vi "York DIHB - Data Capture.vi"() -> ()   [LabVIEW 2020]
doc: "VI used to capture strain gauge data from a Hopskinsons Bar experiment.\n\nOptionally, a calibration (lbs force vs. strain gauge output voltage correlation) can be applied to the measurement data. An interpolation/low pass filter algorith can be used to reduce signal noise.\n\nThe VI uses a queued message handler structure."
uses:
  Typedefs/Messages Cluster - Typedef.ctl
  Typedefs/Program State - Enum.ctl
  Typedefs/GUI Inputs Cluster - Typedef.ctl
  Typedefs/User Event - Enum.ctl
  Typedefs/Program Data - Typedef.ctl
  <vilib>/DAQmx/read.llb/DAQmx Read (Analog 1D Wfm NChan NSamp).vi
  <vilib>/Analysis/5stat.llb/RMS (DBL).vi
  <vilib>/DAQmx/configure/timing.llb/DAQmx Timing (Sample Clock).vi
  <vilib>/DAQmx/configure/trigger.llb/DAQmx Start Trigger (Analog Edge).vi
  <vilib>/DAQmx/miscellaneous.llb/DAQmx Fill In Error Info.vi
  <vilib>/DAQmx/create/channels.llb/DAQmx Create Channel (AI-Voltage-Basic).vi
  <vilib>/Utility/error.llb/Error Cluster From Error Code.vi
  <vilib>/ErrorRing/Error Ring.xnode
  <vilib>/Analysis/NI_AALPro.lvlib
panel:
  out "Projectile Velocity (m/s)":dbl
  out "First Pulse Data":waveform(dbl)(graph)
  out "Gates Graph":waveform(dbl)[](graph)
  out "Strain Gauge Graph":waveform(dbl)(graph)
  out "Warning Icon - Calibration":bool
  out "Warning Icon - Filepath":bool
  in  "Interpolation (Low Pass Filter)":i32
  in  "Calibration File (TXT TSV)":path
  out "File Save Progress":dbl(slide) scale=0.0..100.0
  in  "Filepath to Save Data (TSV)":path
  out "System Ready":bool
  in  "Ready Button":bool
  out "Millions of Samples":dbl
  out "Sample Rate (MHz)":dbl
  in  "Number of Samples":i32=1000000 format="%_3e"
  in  "Sample Rate (Hz)":dbl=2000000.0 format="%_3e"
  # "Instructions\n-Click the run arrow\n-Enter the desired sample rate, the number of samples\n  and the file name.\n-Click Ready\n-Pull the projectile backwards, using the string\n-Clear the impact area\n-Turn on the power switch\n-Push the fire switch\n\nNote: Zero time is time when the fire switch is pressed"
  # "Resolution Increase (bits)"
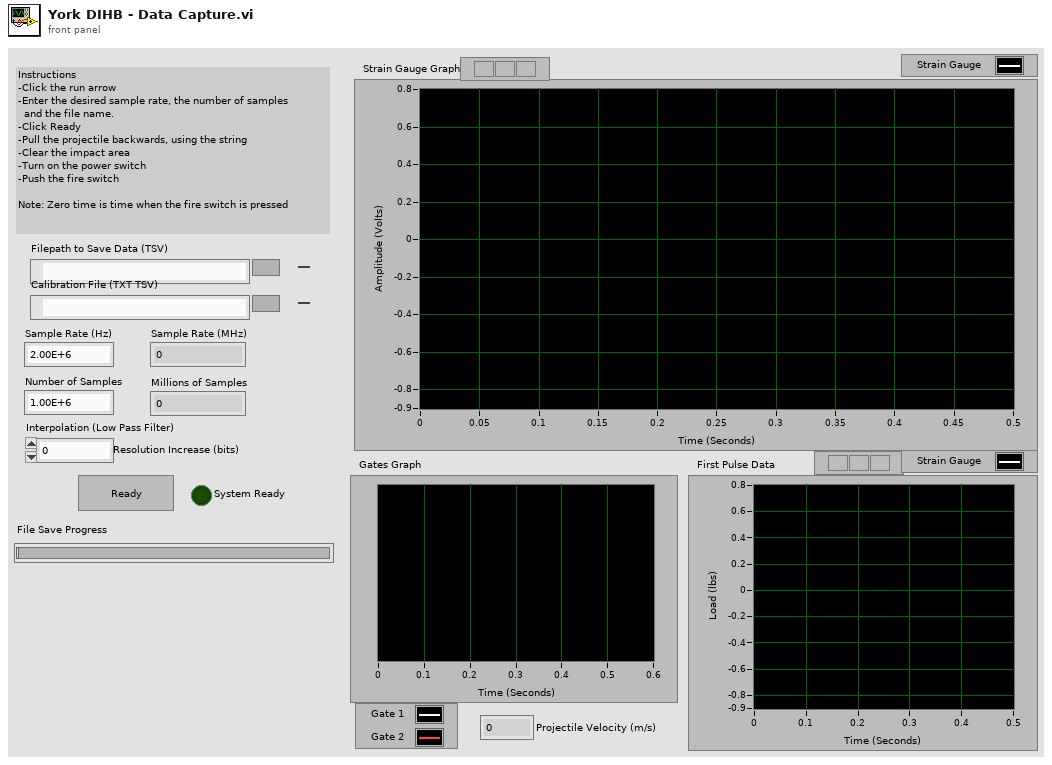
[diagram p1: front panel]
types:
  T1 = typedef "Program Data - Typedef.ctl" = cluster{"DAQmx Task Name":refnum<k21>, "Calibration Y - Load (lbs)":dbl[], "Calibration X - Strain Amplifier (V)":dbl[], "Calibration Slope (lbs/V)":dbl, "Calibration Intercept (lbs)":dbl, "Calibration Error":bool, "Gate 1 (V)":waveform(dbl), "Gate 2 (V)":waveform(dbl), "Strain (V)":waveform(dbl), "Projectile Velocity (m/s)":dbl, "Signal (V)":waveform(dbl), "Noise (V)":waveform(dbl), "Signal to noise ratio":dbl, "Pulse Start Time (ms)":dbl, "Calibrated Signal (lbs)":waveform(dbl), "Filtered Signal (V)":waveform(dbl), "Signal to noise ratio (filtered)":dbl}
  T2 = typedef "User Event - Enum.ctl" = enum16{"Shutdown"}
  T3 = typedef "Program State - Enum.ctl" = enum16{"Make Ready", "Calculate All", "Calculate Velocity", "Calculate Peak Start Time", "Calculate Calibrated Values", "Calculate Filtered Data", "Calculate SNR", "Capture Data", "Download Data", "Load Calibration", "GUI Update", "GUI Show Charts", "GUI Disable Controls", "GUI Enable Controls", "Save Data", "Save Filtered Data", "Save Calibrated Data", "Initialize", "Initialize DAQmx", "Shutdown"}
  T4 = typedef "Messages Cluster - Typedef.ctl" = cluster{"Program State":T3, "GUI Cluster":T5}
  T5 = typedef "GUI Inputs Cluster - Typedef.ctl" = cluster{"Sample Rate (Hz)":dbl, "Number of Samples":i32, "Ready Button":bool, "Filepath to Save Data":path, "Calibration File (TXT TSV)":path, "Interpolation (LP Filter)":dbl}
  T6 = enum8{"Enabled", "Disabled", "Disabled and Grayed Out"}
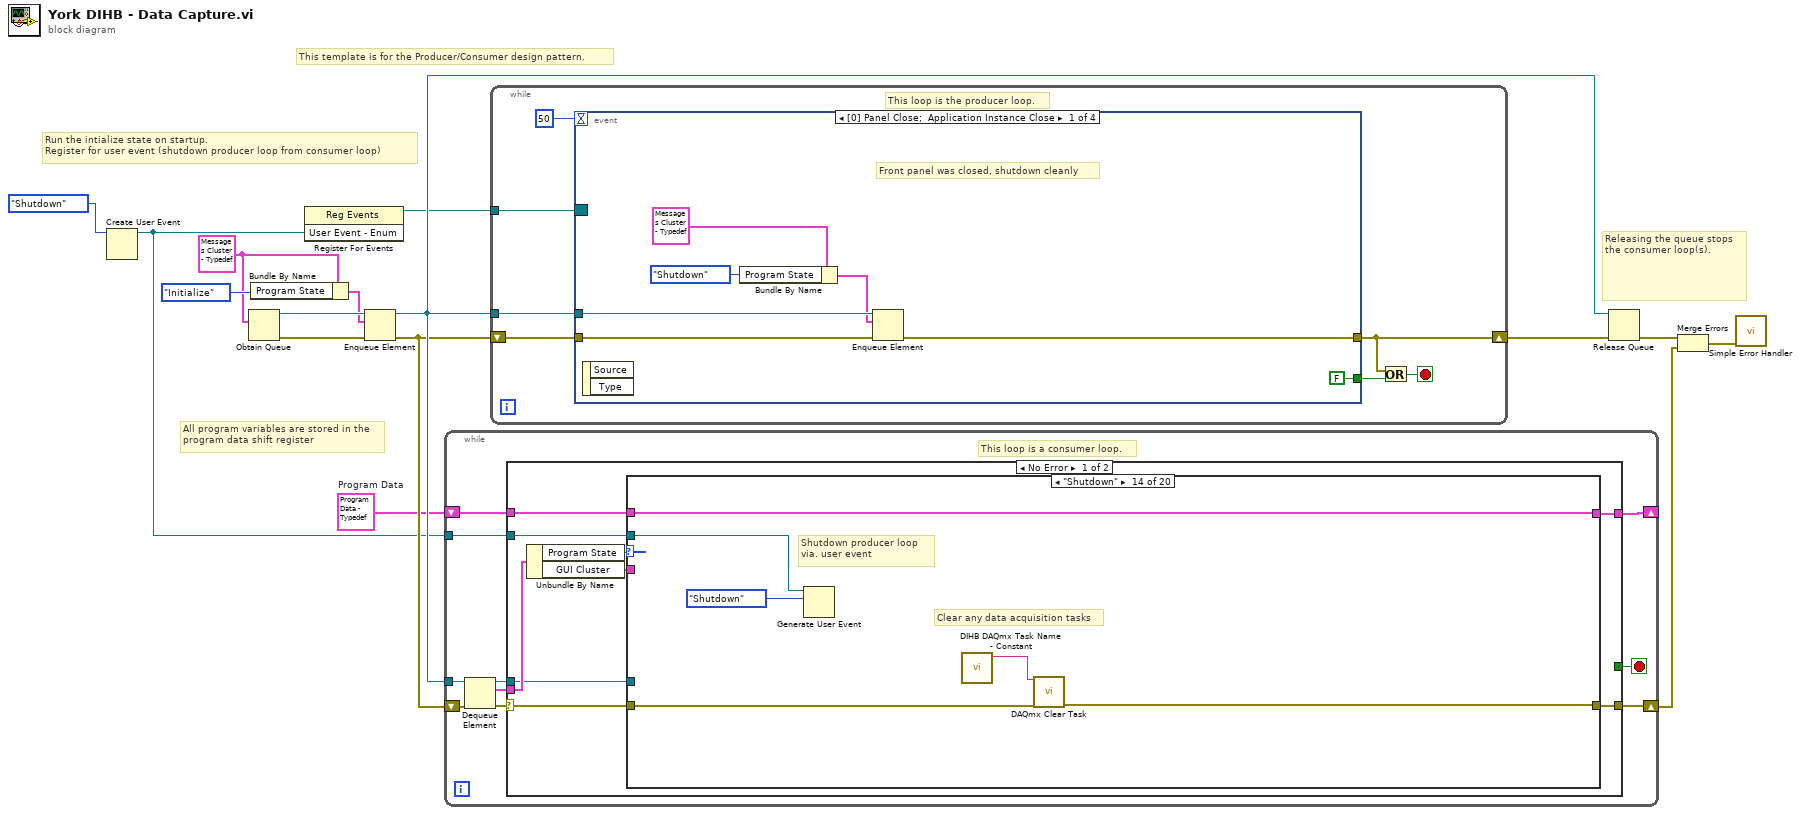
[diagram p0: block diagram]
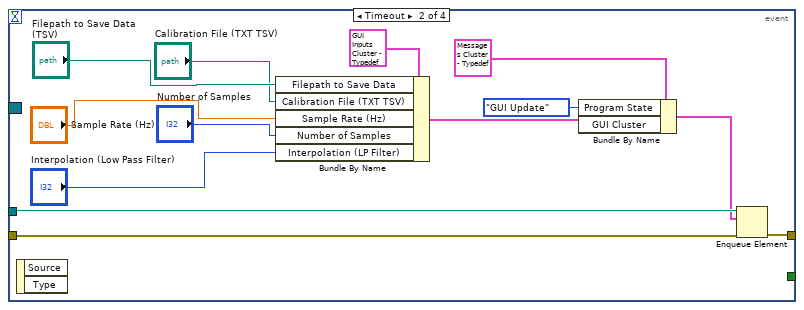
[diagram p2: hidden frame]
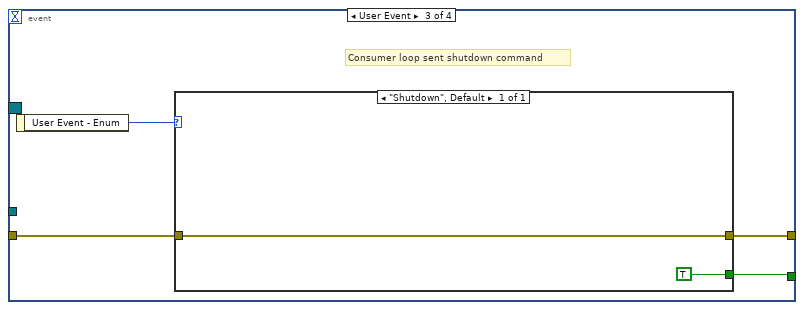
[diagram p3: hidden frame]
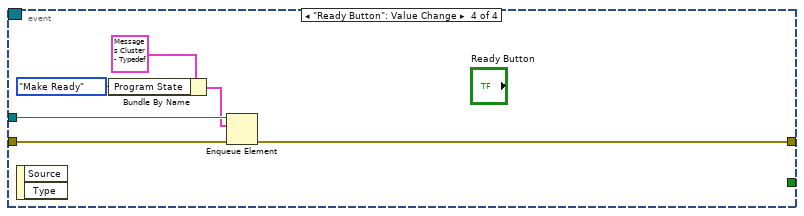
[diagram p4: hidden frame]
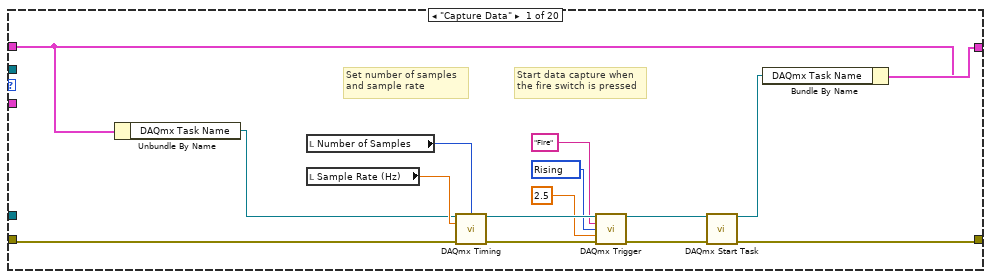
[diagram p5: hidden frame]
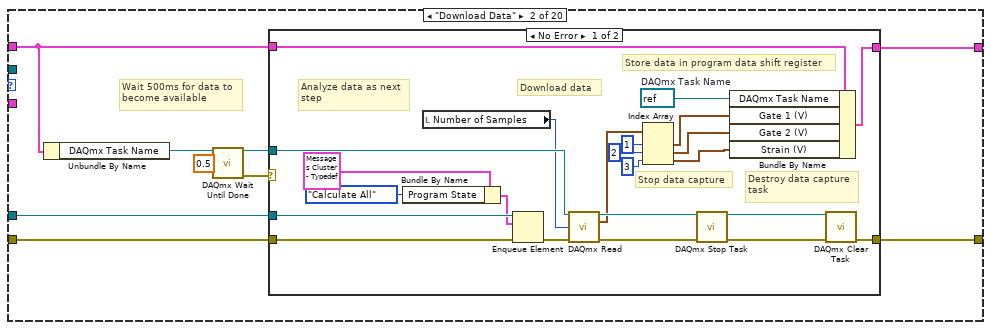
[diagram p6: hidden frame]
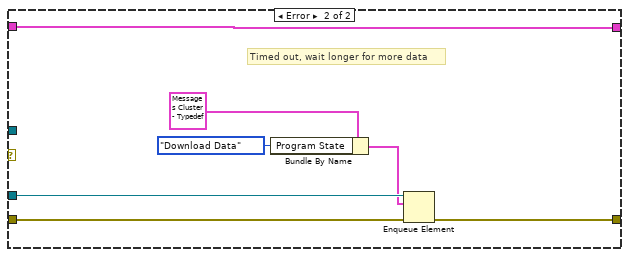
[diagram p7: hidden frame]
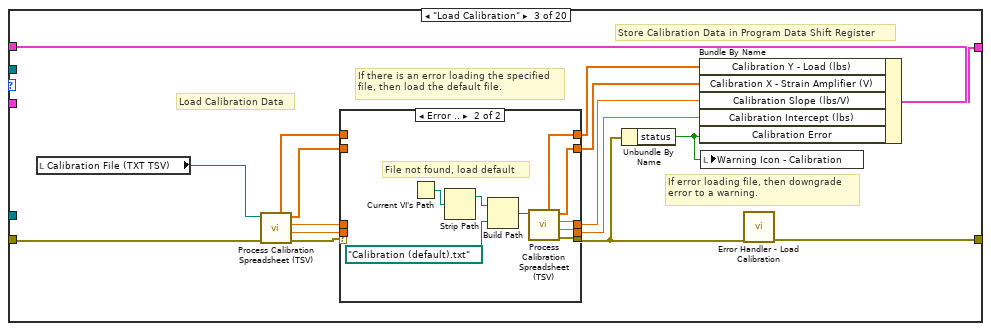
[diagram p8: hidden frame]
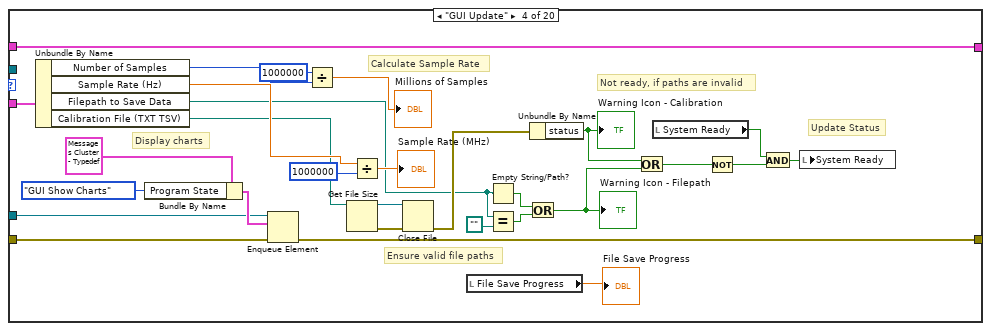
[diagram p10: hidden frame]
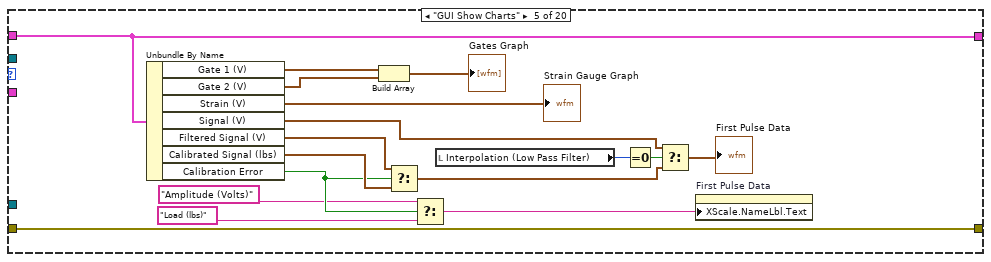
[diagram p11: hidden frame]
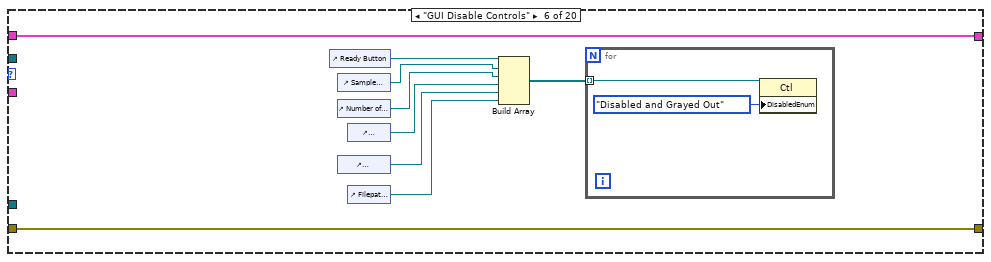
[diagram p12: hidden frame]
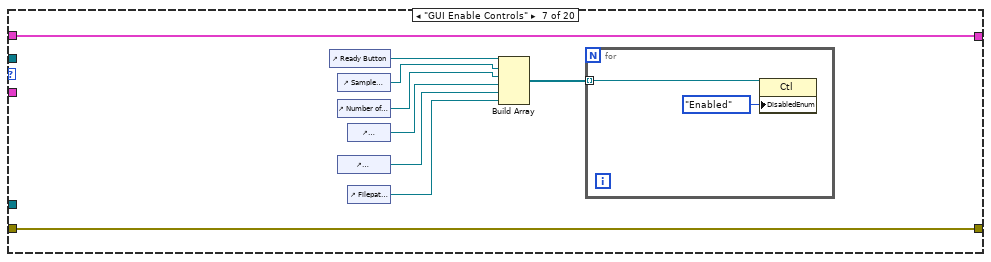
[diagram p13: hidden frame]
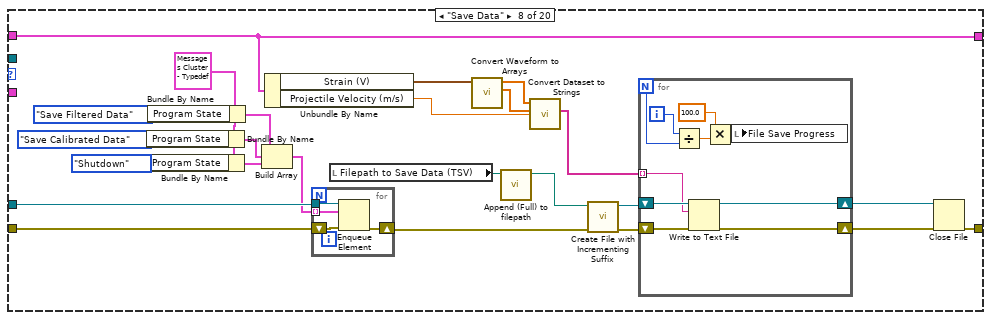
[diagram p14: hidden frame]
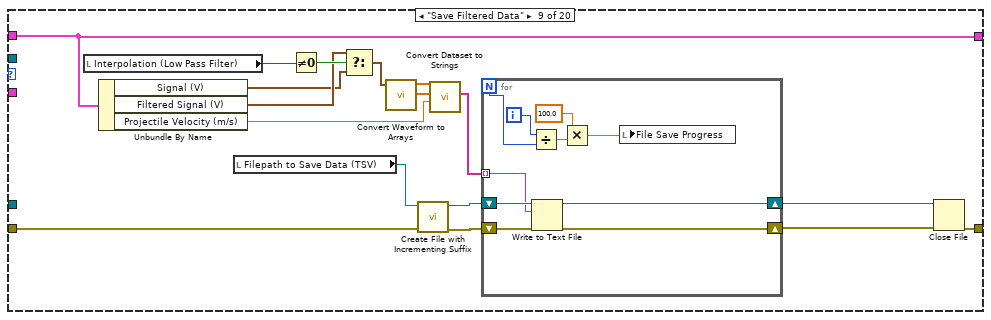
[diagram p15: hidden frame]
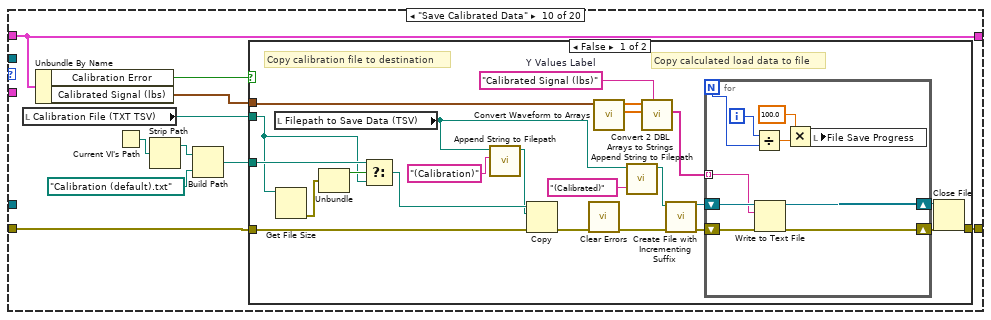
[diagram p16: hidden frame]
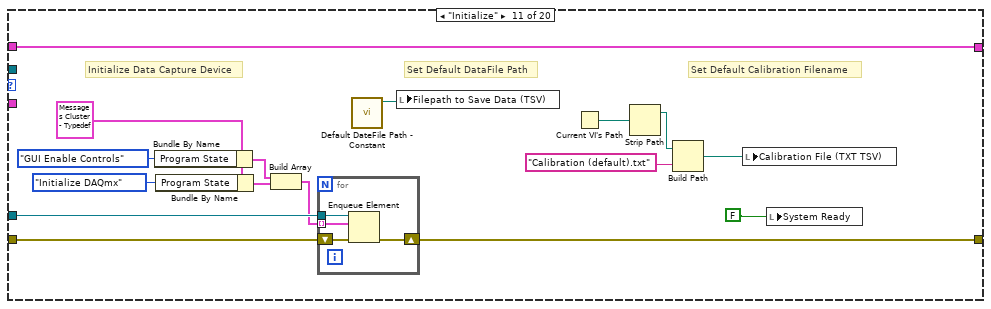
[diagram p18: hidden frame]
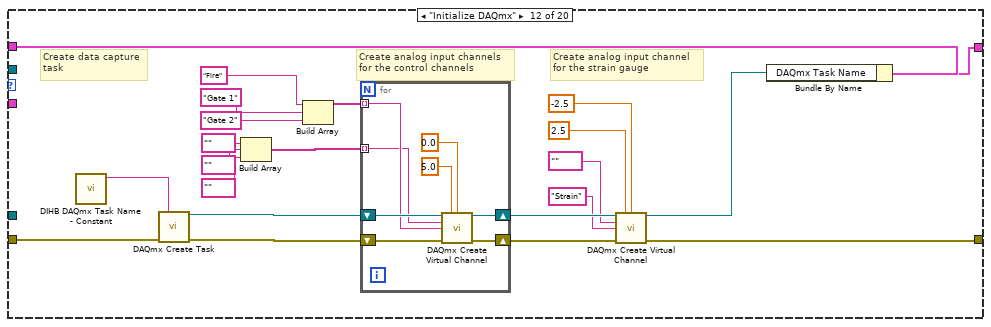
[diagram p19: hidden frame]
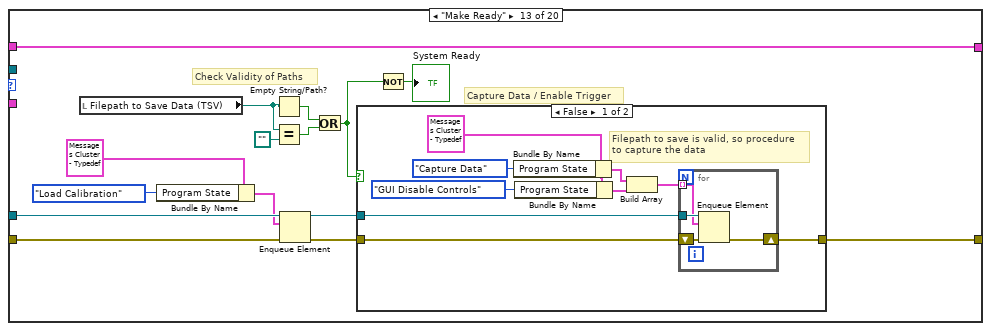
[diagram p20: hidden frame]
diagram:
  w1 = T1 {"DAQmx Task Name"="", "Calibration Y - Load (lbs)"=[], "Calibration X - Strain Amplifier (V)"=[], "Calibration Slope (lbs/V)"=0.0, "Calibration Intercept (lbs)"=0.0, "Calibration Error"=FALSE, "Gate 1 (V)"={"t0"=timestamp(0 s since 1904-01-01), "dt"=1.0, "Y"=[]}, "Gate 2 (V)"={"t0"=timestamp(0 s since 1904-01-01), "dt"=1.0, "Y"=[]}, "Strain (V)"={"t0"=timestamp(0 s since 1904-01-01), "dt"=1.0, "Y"=[]}, "Projectile Velocity (m/s)"=0.0, "Signal (V)"={"t0"=timestamp(0 s since 1904-01-01), "dt"=1.0, "Y"=[]}, "Noise (V)"={"t0"=timestamp(0 s since 1904-01-01), "dt"=1.0, "Y"=[]}, "Signal to noise ratio"=0.0, "Pulse Start Time (ms)"=0.0, "Calibrated Signal (lbs)"={"t0"=timestamp(0 s since 1904-01-01), "dt"=1.0, "Y"=[]}, "Filtered Signal (V)"={"t0"=timestamp(0 s since 1904-01-01), "dt"=1.0, "Y"=[]}, "Signal to noise ratio (filtered)"=0.0}  # Program Data
  w9 = T4 {"Program State"=enum."Calculate Velocity", "GUI Cluster"={"Sample Rate (Hz)"=2000000.0, "Number of Samples"=1000000, "Ready Button"=FALSE, "Filepath to Save Data"=path "", "Calibration File (TXT TSV)"=path "", "Interpolation (LP Filter)"=0.0}} ("input cluster")
  # "All program variables are stored in the\nprogram data shift register"
  # "Run the intialize state on startup.\nRegister for user event (shutdown producer loop from consumer loop)"
  # "Releasing the queue stops the consumer loop(s)."
  # "This template is for the Producer/Consumer design pattern."
  n1 = Create User Event(user event datatype=User_Event_-_Enum."Shutdown" ("User Event - Enum")) -> (user event=w3:refnum<user-event>)  [unwired: 1 in, 1 out]
  n2 = Obtain Queue(element data type=w9) -> (queue out=w13:refnum<queue>, error out=w14:errorcluster)  [unwired: 4 in, 1 out]
  n3 = Bundle By Name(cluster=w9, "Program State"=Program_State_-_Enum."Initialize") -> (w11:T4)
  n4 = register-events(w3) -> (reference out=w4:refnum<event-registration>)  [unwired: 2 in, 1 out]
  n5 = Enqueue Element(queue=w13, element=w11, error in (no error)=w14) -> (queue out=w10:refnum<queue>, error out=w8:errorcluster)  [unwired: 1 in, 1 out]
  n6 = while {
    tunnel: w10 -> [w25]
    shift-right: [w21] -> w6
    shift-left: w8 -> [w20]
    tunnel: w3 -> [w19]
    shift-right: [w16] -> _
    shift-left: w1 -> [w17]
    stop <- w23 stop-if-true
    # "This loop is a consumer loop."
    n7 = Dequeue Element(queue=w25, error in (no error)=w20) -> (queue out=w18:refnum<queue>, element=w22:T4, error out=w24:errorcluster)  [unwired: 1 in, 1 out]
    n8 = case shown="No Error" w24 {
      selector: w24 -> [w31 w484]
      tunnel: w22 -> [w34 _]
      tunnel: [_ TRUE] -> w23
      tunnel: [w30 w484] -> w21
      tunnel: w19 -> [w26 w486]
      tunnel: w18 -> [w29 _]
      tunnel: w17 -> [w28 w483]
      tunnel: [w27 w483] -> w16
      frame No Error {
        n9 = Unbundle By Name(w34) -> ("Program State"=w33:T3, "GUI Cluster"=w32:T5)
        n10 = case shown="\"Shutdown\"" w33 {
          tunnel: w32 -> [_ _ _ w147 _ _ _ _ _ _ _ _ _ _ _ _ _ _ _ _]
          tunnel: w31 -> [w35 w54 w101 w123 w164 w173 w184 w196 w235 w259 w304 w326 w350 w384 w402 w414 w427 w439 w457 w473]
          tunnel: [w45 w53 w99 w121 w164 w173 w184 w198 w236 w260 w303 w321 w355 w383 w401 w411 w426 w438 w457 w473] -> w30
          tunnel: w29 -> [_ w50 _ w122 _ _ _ w194 _ _ w302 _ w352 _ w400 _ _ _ _ _]
          tunnel: w28 -> [w37 w52 w96 w126 w163 w172 w183 w210 w241 w261 w305 w325 w353 w385 w403 w410 w424 w437 w453 w465]
          tunnel: [w39 w51 w95 w126 w163 w172 w183 w210 w241 w261 w305 w324 w353 w385 w403 w409 w423 w436 w452 w464] -> w27
          tunnel: w26 -> [_ _ _ _ _ _ _ _ _ _ _ _ _ w381 _ _ _ _ _ _]
          frame "Capture Data" {
            w43 = 10280 items=["Rising"=10280, "Falling"=10171] ("slope")
            # "Start data capture when\nthe fire switch is pressed"
            # "Set number of samples\nand sample rate"
            n11 = Unbundle By Name(w37) -> ("DAQmx Task Name"=w36:refnum<k21>)
            n12 = local read "Number of Samples"() -> (w40:i32)
            n13 = local read "Sample Rate (Hz)"() -> (w41:dbl)
            n14 = call-poly <vilib>:"DAQmx Timing.vi"("task/channels in"=w36, "samples per channel"=w40, "rate"=w41, "error in"=w35) -> ("task out"=w49:refnum<k21>, "error out"=w46:errorcluster)  [unwired: 10 in]
            n15 = call-poly <vilib>:"DAQmx Trigger.vi"("task/channels in"=w49, "source"="Fire", "slope"=w43, "level"=2.5, "error in"=w46) -> ("task out"=w48:refnum<k21>, "error out"=w47:errorcluster)  [unwired: 9 in]
            n16 = call <vilib>:"DAQmx Start Task.vi"("task/channels in"=w48, "error in"=w47) -> ("task out"=w38:refnum<k21>, "error out"=w45:errorcluster)  [unwired: 12 in]
            n17 = Bundle By Name(cluster=w37, "DAQmx Task Name"=w38) -> (w39:T1)
          }
          frame "Download Data" {
            # "Wait 500ms for data to\nbecome available"
            n18 = Unbundle By Name(w52) -> ("DAQmx Task Name"=w58:refnum<k21>)
            n19 = call <vilib>:"DAQmx Wait Until Done.vi"("task/channels in"=w58, "timeout (sec)"=0.5) -> ("task out"=w56:refnum<k21>, "error out"=w55:errorcluster)  [unwired: 12 in]
            n20 = case shown="No Error" w55 {
              tunnel: w56 -> [w81 _]
              tunnel: w54 -> [w64 w87]
              tunnel: [w78 w85] -> w53
              tunnel: w52 -> [w75 w88]
              tunnel: [w74 w88] -> w51
              tunnel: w50 -> [w62 w86]
              frame No Error {
                w68 = refnum<k21> refnum  # DAQmx Task Name
                # "Analyze data as next\nstep"
                # "Store data in program data shift register"
                # "Destroy data capture\ntask"
                # "Stop data capture"
                # "Download data"
                n21 = Bundle By Name(cluster=T4 {"Program State"=enum."Calculate Velocity", "GUI Cluster"={"Sample Rate (Hz)"=2000000.0, "Number of Samples"=1000000, "Ready Button"=FALSE, "Filepath to Save Data"=path "", "Calibration File (TXT TSV)"=path "", "Interpolation (LP Filter)"=0.0}} ("element"), "Program State"=Program_State_-_Enum."Calculate All") -> (w59:T4)
                n22 = local read "Number of Samples"() -> (w65:i32)
                n23 = Enqueue Element(queue=w62, element=w59, error in (no error)=w64) -> (error out=w63:errorcluster)  [unwired: 1 in, 2 out]
                n24 = call-poly <vilib>:"DAQmx Read.vi"("task/channels in"=w81, "number of samples per channel"=w65, "error in"=w63) -> ("task out"=w77:refnum<k21>, "data"=w73:waveform(dbl)[], "error out"=w80:errorcluster)  [unwired: 10 in]
                n25 = Index Array(array=w73, index #1=1 ("index"), index #2=2 ("index"), index #3=3 ("index")) -> (element #1=w69:waveform(dbl), element #2=w67:waveform(dbl), element #3=w66:waveform(dbl))
                n26 = call <vilib>:"DAQmx Stop Task.vi"("task/channels in"=w77, "error in"=w80) -> ("task out"=w76:refnum<k21>, "error out"=w79:errorcluster)  [unwired: 12 in]
                n27 = Bundle By Name(cluster=w75, "DAQmx Task Name"=w68, "Gate 1 (V)"=w69, "Gate 2 (V)"=w67, "Strain (V)"=w66) -> (w74:T1)
                n28 = call <vilib>:"DAQmx Clear Task.vi"("task in"=w76, "error in"=w79) -> ("error out"=w78:errorcluster)  [unwired: 13 in]
              }
              frame Error {
                # "Timed out, wait longer for more data"
                n29 = Bundle By Name(cluster=T4 {"Program State"=enum."Calculate Velocity", "GUI Cluster"={"Sample Rate (Hz)"=2000000.0, "Number of Samples"=1000000, "Ready Button"=FALSE, "Filepath to Save Data"=path "", "Calibration File (TXT TSV)"=path "", "Interpolation (LP Filter)"=0.0}} ("element"), "Program State"=Program_State_-_Enum."Download Data") -> (w82:T4)
                n30 = Enqueue Element(queue=w86, element=w82, error in (no error)=w87) -> (error out=w85:errorcluster)  [unwired: 1 in, 2 out]
              }
            }
          }
          frame "Load Calibration" {
            # "If there is an error loading the specified\nfile, then load the default file."
            # "If error loading file, then downgrade\nerror to a warning."
            # "Store Calibration Data in Program Data Shift Register"
            # "Load Calibration Data"
            n31 = local read "Calibration File (TXT TSV)"() -> (w100:path)
            n32 = call "Process Calibration Spreadsheet (TSV).vi"("error in"=w101, "Calibration File"=w100) -> ("error out"=w104:errorcluster, "intercept"=w102:dbl, "slope"=w103:dbl, "X - Strain Amplifier (V)"=w97:dbl[], "Y - Load (lbs)"=w98:dbl[])  [unwired: 5 in]
            n33 = case shown="Error .." w104 {
              selector: w104 -> [w109 _]
              tunnel: [w109 w118] -> w94
              tunnel: [w108 w113] -> w92
              tunnel: w103 -> [w108 _]
              tunnel: w102 -> [w107 _]
              tunnel: [w107 w112] -> w93
              tunnel: w98 -> [w106 _]
              tunnel: w97 -> [w105 _]
              tunnel: [w106 w111] -> w90
              tunnel: [w105 w110] -> w91
              frame No Error {
                # "File Found"
              }
              frame Error {
                # "File not found, load default"
                n34 = Current VI's Path() -> (path=w117:path)
                n35 = Strip Path(path=w117) -> (stripped path=w115:path)  [unwired: 1 out]
                n36 = Build Path(base path=w115, name or relative path=path "Calibration (default).txt") -> (appended path=w116:path)
                n37 = call "Process Calibration Spreadsheet (TSV).vi"("Calibration File"=w116) -> ("error out"=w118:errorcluster, "intercept"=w112:dbl, "slope"=w113:dbl, "X - Strain Amplifier (V)"=w110:dbl[], "Y - Load (lbs)"=w111:dbl[])  [unwired: 6 in]
              }
            }
            n38 = Unbundle By Name(w94) -> ("status"=w89:bool)
            n39 = Bundle By Name(cluster=w96, "Calibration Y - Load (lbs)"=w90, "Calibration X - Strain Amplifier (V)"=w91, "Calibration Slope (lbs/V)"=w92, "Calibration Intercept (lbs)"=w93, "Calibration Error"=w89) -> (w95:T1)
            n40 = local write "Warning Icon - Calibration"(w89) -> ()
            n41 = call "Error Handler - Load Calibration.vi"("error in"=w94) -> ("error out"=w99:errorcluster)  [unwired: 10 in]
          }
          frame "GUI Update" {
            # "Display charts"
            # "Not ready, if paths are invalid"
            # "Update Status"
            # "Ensure valid file paths"
            # "Calculate Sample Rate"
            n42 = Unbundle By Name(w147) -> ("Number of Samples"=w146:i32, "Sample Rate (Hz)"=w142:dbl, "Filepath to Save Data"=w133:path, "Calibration File (TXT TSV)"=w140:path)
            n43 = Bundle By Name(cluster=T4 {"Program State"=enum."Calculate Velocity", "GUI Cluster"={"Sample Rate (Hz)"=2000000.0, "Number of Samples"=1000000, "Ready Button"=FALSE, "Filepath to Save Data"=path "", "Calibration File (TXT TSV)"=path "", "Interpolation (LP Filter)"=0.0}} ("element"), "Program State"=Program_State_-_Enum."GUI Show Charts") -> (w125:T4)
            n44 = Enqueue Element(queue=w122, element=w125, error in (no error)=w123) -> (error out=w121:errorcluster)  [unwired: 1 in, 2 out]
            n45 = Divide(x=w146, y=1000000) -> (x/y=→"Millions of Samples":dbl)
            n46 = Get File Size(file=w140) -> (refnum out=w138:refnum<file>, 0:w139:errorcluster)  [unwired: 1 in, 1 out]
            n47 = Divide(x=w142, y=1000000) -> (x/y=→"Sample Rate (MHz)":dbl)
            n48 = Close File(refnum=w138, error in=w139) -> (error out=w137:errorcluster)  [unwired: 1 out]
            n49 = local read "File Save Progress"() -> (→"File Save Progress":dbl)
            n50 = Empty String/Path?(string/path=w133) -> (empty?=w134:bool)
            n51 = Equal?(x=w133, y=path "") -> (x = y?=w135:bool)
            n52 = Or(x=w134, y=w135) -> (x .or. y?=w131:bool)
            "Warning Icon - Filepath" <- w131
            n53 = Unbundle By Name(w137) -> ("status"=w132:bool)
            "Warning Icon - Calibration" <- w132
            n54 = Or(x=w132, y=w131) -> (x .or. y?=w128:bool)
            n55 = local read "System Ready"() -> (w130:bool)
            n56 = Not(x=w128) -> (.not. x?=w129:bool)
            n57 = And(x=w130, y=w129) -> (x .and. y?=w127:bool)
            n58 = local write "System Ready"(w127) -> ()
          }
          frame "GUI Show Charts" {
            n59 = Unbundle By Name(w163) -> ("Gate 1 (V)"=w162:waveform(dbl), "Gate 2 (V)"=w161:waveform(dbl), "Strain (V)"=→"Strain Gauge Graph":waveform(dbl), "Signal (V)"=w155:waveform(dbl), "Filtered Signal (V)"=w158:waveform(dbl), "Calibrated Signal (lbs)"=w152:waveform(dbl), "Calibration Error"=w151:bool)
            n60 = Build Array(w162, w161) -> (→"Gates Graph":waveform(dbl)[])
            n61 = Select(t=w158, s=w151, f=w152) -> (s? t:f=w154:waveform(dbl))
            n62 = Select(t="Amplitude (Volts)", s=w151, f="Load (lbs)") -> (s? t:f=w148:string)
            n63 = local read "Interpolation (Low Pass Filter)"() -> (w156:i32)
            n64 = Equal To 0?(x=w156) -> (x = 0?=w157:bool)
            n65 = Select(t=w155, s=w157, f=w154) -> (s? t:f=→"First Pulse Data":waveform(dbl))
            n66 = property on="First Pulse Data" class="WFGraph (strict)"("XScale.NameLbl.Text"=w148) -> ()  [unwired: 2 in, 2 out]
          }
          frame "GUI Disable Controls" {
            n67 = control-ref of="Ready Button"() -> (w171:refnum<vi>)
            n68 = control-ref of="Sample Rate (Hz)"() -> (w170:refnum<vi>)
            n69 = control-ref of="Number of Samples"() -> (w169:refnum<vi>)
            n70 = control-ref of="Interpolation (Low Pass Filter)"() -> (w167:refnum<vi>)
            n71 = control-ref of="Calibration File (TXT TSV)"() -> (w168:refnum<vi>)
            n72 = control-ref of="Filepath to Save Data (TSV)"() -> (w166:refnum<vi>)
            n73 = Build Array(w171, w170, w169, w168, w167, w166) -> (w165:refnum<vi>[])
            n74 = for {
              tunnel: w165 -> [w175] mode=indexing
              n75 = property class="Ctl"(reference=w175, "DisabledEnum"=T6."Disabled and Grayed Out" ("Disabled")) -> ()  [unwired: 1 in, 2 out]
            }
          }
          frame "GUI Enable Controls" {
            n76 = control-ref of="Ready Button"() -> (w182:refnum<vi>)
            n77 = control-ref of="Sample Rate (Hz)"() -> (w181:refnum<vi>)
            n78 = control-ref of="Number of Samples"() -> (w180:refnum<vi>)
            n79 = control-ref of="Interpolation (Low Pass Filter)"() -> (w178:refnum<vi>)
            n80 = control-ref of="Calibration File (TXT TSV)"() -> (w179:refnum<vi>)
            n81 = control-ref of="Filepath to Save Data (TSV)"() -> (w177:refnum<vi>)
            n82 = Build Array(w182, w181, w180, w179, w178, w177) -> (w176:refnum<vi>[])
            n83 = for {
              tunnel: w176 -> [w186] mode=indexing
              n84 = property class="Ctl"(reference=w186, "DisabledEnum"=T6."Enabled" ("Disabled")) -> ()  [unwired: 1 in, 2 out]
            }
          }
          frame "Save Data" {
            w191 = T4 {"Program State"=enum."Calculate Velocity", "GUI Cluster"={"Sample Rate (Hz)"=2000000.0, "Number of Samples"=1000000, "Ready Button"=FALSE, "Filepath to Save Data"=path "", "Calibration File (TXT TSV)"=path "", "Interpolation (LP Filter)"=0.0}} ("input cluster")
            n85 = Bundle By Name(cluster=w191, "Program State"=Program_State_-_Enum."Save Calibrated Data") -> (w189:T4)
            n86 = Bundle By Name(cluster=w191, "Program State"=Program_State_-_Enum."Shutdown") -> (w190:T4)
            n87 = Bundle By Name(cluster=w191, "Program State"=Program_State_-_Enum."Save Filtered Data") -> (w188:T4)
            n88 = Build Array(w188, w189, w190) -> (w187:T4[])
            n89 = Unbundle By Name(w210) -> ("Strain (V)"=w209:waveform(dbl), "Projectile Velocity (m/s)"=w208:dbl)
            n90 = for {
              tunnel: w194 -> [w212]
              shift-right: [w213] -> w195
              shift-left: w196 -> [w214]
              tunnel: w187 -> [w211] mode=indexing
              n91 = Enqueue Element(queue=w212, element=w211, error in (no error)=w214) -> (error out=w213:errorcluster)  [unwired: 1 in, 2 out]
            }
            n92 = local read "Filepath to Save Data (TSV)"() -> (w201:path)
            n93 = call "Convert Waveform to Arrays.vi"("Waveform In"=w209) -> ("X Values (Seconds)"=w206:dbl[], "Y Values (Voltage)"=w207:dbl[])  [unwired: 9 in]
            n94 = call "Append (Full) to filepath.vi"("Filepath to Save Data"=w201) -> ("appended path"=w203:path)  [unwired: 10 in]
            n95 = call "Convert Dataset to Strings.vi"("Projectile Velocity (Meters/Second)"=w208, "X Values (Seconds)"=w206, "Y Values (Voltage)"=w207) -> ("DataSet Rows"=w202:string[])  [unwired: 8 in]
            n96 = call <vilib>:"Create File with Incrementing Suffix.vi"("error in (no error)"=w195, "file path"=w203) -> ("error out"=w205:errorcluster, "refnum out"=w204:refnum<file>)  [unwired: 7 in, 1 out]
            n97 = for {
              N -> [w218]
              shift-right: [w224] -> w200
              shift-left: w205 -> [w222]
              shift-right: [w223] -> w199
              shift-left: w204 -> [w221]
              tunnel: w202 -> [w220] mode=indexing
              i -> [w219]
              n98 = Divide(x=w219, y=w218) -> (x/y=w217:dbl)
              n99 = Write to Text File(file (use dialog)=w221, text=w220, error in=w222) -> (refnum out=w223:refnum<file>, error out=w224:errorcluster)  [unwired: 1 in, 1 out]
              n100 = Multiply(x=100.0, y=w217) -> (x*y=w215:dbl)
              n101 = local write "File Save Progress"(w215) -> ()
            }
            n102 = Close File(refnum=w199, error in=w200) -> (error out=w198:errorcluster)  [unwired: 1 out]
          }
          frame "Save Filtered Data" {
            n103 = local read "Interpolation (Low Pass Filter)"() -> (w234:i32)
            n104 = Unbundle By Name(w241) -> ("Signal (V)"=w231:waveform(dbl), "Filtered Signal (V)"=w232:waveform(dbl), "Projectile Velocity (m/s)"=w226:dbl)
            n105 = local read "Filepath to Save Data (TSV)"() -> (w229:path)
            n106 = Not Equal To 0?(x=w234) -> (x != 0?=w233:bool)
            n107 = Select(t=w232, s=w233, f=w231) -> (s? t:f=w230:waveform(dbl))
            n108 = call "Convert Waveform to Arrays.vi"("Waveform In"=w230) -> ("X Values (Seconds)"=w227:dbl[], "Y Values (Voltage)"=w228:dbl[])  [unwired: 9 in]
            n109 = call <vilib>:"Create File with Incrementing Suffix.vi"("error in (no error)"=w235, "file path"=w229) -> ("error out"=w240:errorcluster, "refnum out"=w239:refnum<file>)  [unwired: 7 in, 1 out]
            n110 = call "Convert Dataset to Strings.vi"("Projectile Velocity (Meters/Second)"=w226, "X Values (Seconds)"=w227, "Y Values (Voltage)"=w228) -> ("DataSet Rows"=w225:string[])  [unwired: 8 in]
            n111 = for {
              N -> [w245]
              shift-right: [w251] -> w238
              shift-left: w240 -> [w249]
              shift-right: [w250] -> w237
              shift-left: w239 -> [w248]
              tunnel: w225 -> [w247] mode=indexing
              i -> [w246]
              n112 = Divide(x=w246, y=w245) -> (x/y=w244:dbl)
              n113 = Write to Text File(file (use dialog)=w248, text=w247, error in=w249) -> (refnum out=w250:refnum<file>, error out=w251:errorcluster)  [unwired: 1 in, 1 out]
              n114 = Multiply(x=100.0, y=w244) -> (x*y=w242:dbl)
              n115 = local write "File Save Progress"(w242) -> ()
            }
            n116 = Close File(refnum=w237, error in=w238) -> (error out=w236:errorcluster)  [unwired: 1 out]
          }
          frame "Save Calibrated Data" {
            n117 = local read "Calibration File (TXT TSV)"() -> (w253:path)
            n118 = Unbundle By Name(w261) -> ("Calibration Error"=w257:bool, "Calibrated Signal (lbs)"=w258:waveform(dbl))
            n119 = Current VI's Path() -> (path=w256:path)
            n120 = Strip Path(path=w256) -> (stripped path=w255:path)  [unwired: 1 out]
            n121 = Build Path(base path=w255, name or relative path=path "Calibration (default).txt") -> (appended path=w252:path)
            n122 = case shown="False" w257 {
              tunnel: [w280 w295] -> w260
              tunnel: w259 -> [w264 w295]
              tunnel: w258 -> [w277 _]
              tunnel: w253 -> [w269 _]
              tunnel: w252 -> [w270 _]
              frame False {
                w273 = "Calibrated Signal (lbs)"  # Y Values Label
                # "Copy calculated load data to file"
                # "Copy calibration file to destination"
                n123 = local read "Filepath to Save Data (TSV)"() -> (w267:path)
                n124 = Get File Size(file=w269) -> (0:w272:errorcluster)  [unwired: 1 in, 2 out]
                n125 = Unbundle(w272) -> ("status"=w271:bool)  [unwired: 2 out]
                n126 = Select(t=w270, s=w271, f=w269) -> (s? t:f=w268:path)
                n127 = call "Append String to Filepath.vi"("Append"="(Calibration)", "Filepath to Save Data"=w267) -> ("appended path"=w266:path)  [unwired: 9 in]
                n128 = Copy(8:w264, 10:w266, 11:w268) -> (0:w263:errorcluster)  [unwired: 2 in, 2 out]
                n129 = call <vilib>:"Clear Errors.vi"("error in (no error)"=w263) -> ("error out"=w262:errorcluster)  [unwired: 5 in, 1 out]
                n130 = call "Convert Waveform to Arrays.vi"("Waveform In"=w277) -> ("X Values (Seconds)"=w275:dbl[], "Y Values (Voltage)"=w276:dbl[])  [unwired: 9 in]
                n131 = call "Append String to Filepath.vi"("Append"="(Calibrated)", "Filepath to Save Data"=w267) -> ("appended path"=w279:path)  [unwired: 9 in]
                n132 = call "Convert 2 DBL Arrays to Strings.vi"("Y Values Label"=w273, "X Values (Seconds)"=w275, "Y Values (Voltage)"=w276) -> ("DataSet Rows"=w274:string[])  [unwired: 8 in]
                n133 = call <vilib>:"Create File with Incrementing Suffix.vi"("error in (no error)"=w262, "file path"=w279) -> ("error out"=w284:errorcluster, "refnum out"=w283:refnum<file>)  [unwired: 7 in, 1 out]
                n134 = for {
                  N -> [w288]
                  shift-right: [w294] -> w282
                  shift-left: w284 -> [w292]
                  shift-right: [w293] -> w281
                  shift-left: w283 -> [w291]
                  tunnel: w274 -> [w290] mode=indexing
                  i -> [w289]
                  n135 = Divide(x=w289, y=w288) -> (x/y=w287:dbl)
                  n136 = Write to Text File(file (use dialog)=w291, text=w290, error in=w292) -> (refnum out=w293:refnum<file>, error out=w294:errorcluster)  [unwired: 1 in, 1 out]
                  n137 = Multiply(x=100.0, y=w287) -> (x*y=w285:dbl)
                  n138 = local write "File Save Progress"(w285) -> ()
                }
                n139 = Close File(refnum=w281, error in=w282) -> (error out=w280:errorcluster)  [unwired: 1 out]
              }
              frame True {
                # "Error loading calibration data, so don't save anything"
              }
            }
          }
          frame "Initialize" {
            w299 = T4 {"Program State"=enum."Calculate Velocity", "GUI Cluster"={"Sample Rate (Hz)"=2000000.0, "Number of Samples"=1000000, "Ready Button"=FALSE, "Filepath to Save Data"=path "", "Calibration File (TXT TSV)"=path "", "Interpolation (LP Filter)"=0.0}} ("element")
            # "Initialize Data Capture Device"
            # "Set Default DataFile Path"
            # "Set Default Calibration Filename"
            n140 = Bundle By Name(cluster=w299, "Program State"=Program_State_-_Enum."GUI Enable Controls") -> (w297:T4)
            n141 = Bundle By Name(cluster=w299, "Program State"=Program_State_-_Enum."Initialize DAQmx") -> (w298:T4)
            n142 = Build Array(w297, w298) -> (w296:T4[])
            n143 = for {
              tunnel: w302 -> [w313]
              shift-right: [w314] -> w303
              shift-left: w304 -> [w315]
              tunnel: w296 -> [w312] mode=indexing
              n144 = Enqueue Element(queue=w313, element=w312, error in (no error)=w315) -> (error out=w314:errorcluster)  [unwired: 1 in, 2 out]
            }
            n145 = call "Default DateFile Path - Constant.vi"() -> ("Datafile Path (Default)"=w311:path)  [unwired: 11 in]
            n146 = local write "Filepath to Save Data (TSV)"(w311) -> ()
            n147 = Current VI's Path() -> (path=w310:path)
            n148 = Strip Path(path=w310) -> (stripped path=w309:path)  [unwired: 1 out]
            n149 = Build Path(base path=w309, name or relative path="Calibration (default).txt" ("string")) -> (appended path=w308:path)
            n150 = local write "Calibration File (TXT TSV)"(w308) -> ()
            n151 = local write "System Ready"(FALSE ("System Ready")) -> ()
          }
          frame "Initialize DAQmx" {
            # "Create analog input channel\nfor the strain gauge"
            # "Create data capture\ntask"
            # "Create analog input channels\nfor the control channels"
            n152 = call "DIHB DAQmx Task Name - Constant.vi"() -> ("DIHB DAQmx Task Name"=w333:string)  [unwired: 11 in]
            n153 = call <vilib>:"DAQmx Create Task.vi"("new task name"=w333, "error in"=w326) -> ("task out"=w334:refnum<k21>, "error out"=w332:errorcluster)  [unwired: 12 in]
            n154 = Build Array(tag "" ("physical channels"), tag "" ("physical channels"), tag "" ("physical channels")) -> (w330:tag[])
            n155 = Build Array("Fire", "Gate 1", "Gate 2") -> (w331:string[])
            n156 = for {
              shift-right: [w345] -> w323
              shift-left: w334 -> [w341]
              shift-right: [w344] -> w322
              shift-left: w332 -> [w340]
              tunnel: w331 -> [w339] mode=indexing
              tunnel: w330 -> [w338] mode=indexing
              n157 = call-poly <vilib>:"DAQmx Create Virtual Channel.vi"("task in"=w341, "maximum value"=5.0, "minimum value"=0.0, "physical channels"=w338, "name to assign"=w339, "error in"=w340) -> ("task out"=w345:refnum<k21>, "error out"=w344:errorcluster)  [unwired: 8 in]
            }
            n158 = call-poly <vilib>:"DAQmx Create Virtual Channel.vi"("task in"=w323, "maximum value"=2.5, "minimum value"=-2.5, "physical channels"=tag "", "name to assign"="Strain", "error in"=w322) -> ("task out"=w320:refnum<k21>, "error out"=w321:errorcluster)  [unwired: 8 in]
            n159 = Bundle By Name(cluster=w325, "DAQmx Task Name"=w320) -> (w324:T1)
          }
          frame "Make Ready" {
            # "Capture Data / Enable Trigger"
            # "Check Validity of Paths"
            n160 = local read "Filepath to Save Data (TSV)"() -> (w357:path)
            n161 = Bundle By Name(cluster=T4 {"Program State"=enum."Calculate Velocity", "GUI Cluster"={"Sample Rate (Hz)"=2000000.0, "Number of Samples"=1000000, "Ready Button"=FALSE, "Filepath to Save Data"=path "", "Calibration File (TXT TSV)"=path "", "Interpolation (LP Filter)"=0.0}} ("element"), "Program State"=Program_State_-_Enum."Load Calibration") -> (w346:T4)
            n162 = Empty String/Path?(string/path=w357) -> (empty?=w358:bool)
            n163 = Equal?(x=w357, y=path "") -> (x = y?=w359:bool)
            n164 = Enqueue Element(queue=w352, element=w346, error in (no error)=w350) -> (queue out=w351:refnum<queue>, error out=w349:errorcluster)  [unwired: 1 in, 1 out]
            n165 = Or(x=w358, y=w359) -> (x .or. y?=w356:bool)
            n166 = case shown="False" w356 {
              tunnel: [w368 w374] -> w355
              tunnel: w349 -> [w369 _]
              tunnel: w351 -> [w366 _]
              frame False {
                w364 = T4 {"Program State"=enum."Calculate Velocity", "GUI Cluster"={"Sample Rate (Hz)"=2000000.0, "Number of Samples"=1000000, "Ready Button"=FALSE, "Filepath to Save Data"=path "", "Calibration File (TXT TSV)"=path "", "Interpolation (LP Filter)"=0.0}} ("element")
                # "Filepath to save is valid, so procedure\nto capture the data"
                n167 = Bundle By Name(cluster=w364, "Program State"=Program_State_-_Enum."Capture Data") -> (w362:T4)
                n168 = Bundle By Name(cluster=w364, "Program State"=Program_State_-_Enum."GUI Disable Controls") -> (w363:T4)
                n169 = Build Array(w362, w363) -> (w361:T4[])
                n170 = for {
                  tunnel: w366 -> [w371]
                  shift-right: [w372] -> w368
                  shift-left: w369 -> [w373]
                  tunnel: w361 -> [w370] mode=indexing
                  n171 = Enqueue Element(queue=w371, element=w370, error in (no error)=w373) -> (error out=w372:errorcluster)  [unwired: 1 in, 2 out]
                }
              }
              frame True {
                # "Error encountered, don't make ready"
                n172 = xnode "Error Ring"() -> ("error out"=w374:errorcluster)
              }
            }
            n173 = Not(x=w356) -> (.not. x?=→"System Ready":bool)
          }
          frame "Shutdown" {
            # "Clear any data acquisition tasks"
            # "Shutdown producer loop\nvia. user event"
            n174 = Generate User Event(user event=w381, event data cluster=User_Event_-_Enum."Shutdown" ("event data")) -> ()  [unwired: 2 in, 2 out]
            n175 = call "DIHB DAQmx Task Name - Constant.vi"() -> ("DIHB DAQmx Task Name"=w382:string)  [unwired: 11 in]
            n176 = call <vilib>:"DAQmx Clear Task.vi"("task in"=w382, "error in"=w384) -> ("error out"=w383:errorcluster)  [unwired: 13 in]
          }
          frame "Calculate All" {
            w388 = T4 {"Program State"=enum."Calculate Velocity", "GUI Cluster"={"Sample Rate (Hz)"=2000000.0, "Number of Samples"=1000000, "Ready Button"=FALSE, "Filepath to Save Data"=path "", "Calibration File (TXT TSV)"=path "", "Interpolation (LP Filter)"=0.0}} ("element")
            n177 = Bundle By Name(cluster=w388, "Program State"=Program_State_-_Enum."Calculate Velocity") -> (w395:T4)
            n178 = Bundle By Name(cluster=w388, "Program State"=Program_State_-_Enum."Calculate Peak Start Time") -> (w394:T4)
            n179 = Bundle By Name(cluster=w388, "Program State"=Program_State_-_Enum."Calculate Filtered Data") -> (w393:T4)
            n180 = Bundle By Name(cluster=w388, "Program State"=Program_State_-_Enum."Calculate Calibrated Values") -> (w391:T4)
            n181 = Bundle By Name(cluster=w388, "Program State"=Program_State_-_Enum."Save Data") -> (w386:T4)
            n182 = Bundle By Name(cluster=w388, "Program State"=Program_State_-_Enum."Calculate SNR") -> (w389:T4)
            n183 = Build Array(w395, w394, w393, w391, w389, w386) -> (w396:T4[])
            n184 = for {
              tunnel: w400 -> [w405]
              shift-right: [w406] -> w401
              shift-left: w402 -> [w407]
              tunnel: w396 -> [w404] mode=indexing
              n185 = Enqueue Element(queue=w405, element=w404, error in (no error)=w407) -> (error out=w406:errorcluster)  [unwired: 1 in, 2 out]
            }
          }
          frame "Calculate Velocity", Default {
            n186 = Unbundle By Name(w410) -> ("Gate 2 (V)"=w416:waveform(dbl), "Gate 1 (V)"=w415:waveform(dbl))
            n187 = call "Calculate Trigger Time (Falling Edge).vi"("Waveform In"=w415) -> ("error out"=w412:errorcluster, "Trigger Time (Seconds)"=w418:dbl)  [unwired: 7 in, 2 out]
            n188 = call "Calculate Trigger Time (Falling Edge).vi"("Waveform In"=w416) -> ("error out"=w413:errorcluster, "Trigger Time (Seconds)"=w417:dbl)  [unwired: 7 in, 2 out]
            n189 = call "Distance Between Gates - Constant.vi"() -> ("Distance Between Gates (m)"=w419:dbl)  [unwired: 11 in]
            n190 = Merge Errors(w413, w412, w414) -> (w411:errorcluster)
            n191 = Subtract(x=w417, y=w418) -> (x-y=w420:dbl)
            n192 = Divide(x=w419, y=w420) -> (x/y=w408:dbl)
            "Projectile Velocity (m/s)" <- w408
            n193 = Bundle By Name(cluster=w410, "Projectile Velocity (m/s)"=w408) -> (w409:T1)
          }
          frame "Calculate Peak Start Time" {
            n194 = Unbundle By Name(w424) -> ("Strain (V)"=w425:waveform(dbl))
            n195 = call "Identify Pulse and Noise.vi"("error in"=w427, "Waveform In"=w425) -> ("error out"=w426:errorcluster, "Signal Waveform Out"=w421:waveform(dbl), "Noise Waveform Out"=w422:waveform(dbl))  [unwired: 5 in, 2 out]
            n196 = Bundle By Name(cluster=w424, "Signal (V)"=w421, "Noise (V)"=w422) -> (w423:T1)
          }
          frame "Calculate Calibrated Values" {
            n197 = local read "Interpolation (Low Pass Filter)"() -> (w428:i32)
            n198 = Unbundle By Name(w437) -> ("Filtered Signal (V)"=w431:waveform(dbl), "Signal (V)"=w430:waveform(dbl), "Calibration Slope (lbs/V)"=w434:dbl, "Calibration Intercept (lbs)"=w435:dbl, "Calibration Error"=w441:bool)
            n199 = Not Equal To 0?(x=w428) -> (x != 0?=w429:bool)
            n200 = Select(t=w431, s=w429, f=w430) -> (s? t:f=w432:waveform(dbl))
            n201 = Bundle(cluster=errorcluster {"status"=FALSE, "code"=0, "source"=""} ("error constant"), "status"=w441) -> (w440:errorcluster)  [unwired: 2 in]
            n202 = case shown="No Error" w440 {
              tunnel: w439 -> [w448 w450]
              tunnel: [w448 w450] -> w438
              tunnel: w432 -> [w446 _]
              tunnel: w435 -> [w444 _]
              tunnel: w434 -> [w445 _]
              tunnel: [w443 waveform(dbl) {"t0"=timestamp(0 s since 1904-01-01), "dt"=1.0, "Y"=[]} ("Waveform")] -> w433
              frame No Error {
                n203 = Multiply(x=w446, y=w445) -> (x*y=w447:waveform(dbl))
                n204 = Add(x=w444, y=w447) -> (x+y=w443:waveform(dbl))
              }
              frame Error {
              }
            }
            n205 = Bundle By Name(cluster=w437, "Calibrated Signal (lbs)"=w433) -> (w436:T1)
          }
          frame "Calculate Filtered Data" {
            n206 = Unbundle By Name(w453) -> ("Signal (V)"=w456:waveform(dbl))
            n207 = local read "Interpolation (Low Pass Filter)"() -> (w454:i32)
            n208 = Not Equal To 0?(x=w454) -> (x != 0?=w455:bool)
            n209 = case shown="True" w455 {
              tunnel: [waveform(dbl) {"t0"=timestamp(0 s since 1904-01-01), "dt"=1.0, "Y"=[]} ("Waveform") w459] -> w451
              tunnel: w456 -> [_ w461]
              tunnel: w454 -> [_ w460]
              frame False {
              }
              frame True {
                n210 = call "Interpolate Oversampled Data.vi"("Bits of Precision Increase"=w460, "Waveform in"=w461) -> ("Waveform out"=w459:waveform(dbl))  [unwired: 9 in]
              }
            }
            n211 = Bundle By Name(cluster=w453, "Filtered Signal (V)"=w451) -> (w452:T1)
          }
          frame "Calculate SNR" {
            n212 = Unbundle By Name(w465) -> ("Signal (V)"=w472:waveform(dbl), "Noise (V)"=w467:waveform(dbl), "Filtered Signal (V)"=w469:waveform(dbl))
            n213 = local read "Interpolation (Low Pass Filter)"() -> (w466:i32)
            n214 = call-poly <vilib>:"RMS.vi"("X"=w472) -> ("rms value"=w471:dbl)  [unwired: 1 out]
            n215 = call-poly <vilib>:"RMS.vi"("X"=w467) -> ("rms value"=w470:dbl)  [unwired: 1 out]
            n216 = Divide(x=w471, y=w470) -> (x/y=w462:dbl)
            n217 = Not Equal To 0?(x=w466) -> (x != 0?=w468:bool)
            n218 = case shown="True" w468 {
              tunnel: w469 -> [_ w481]
              tunnel: w467 -> [_ w480]
              tunnel: w466 -> [_ w479]
              tunnel: [0.0 w475] -> w463
              frame False {
              }
              frame True {
                n219 = call-poly <vilib>:"RMS.vi"("X"=w481) -> ("rms value"=w476:dbl)  [unwired: 1 out]
                n220 = call "Interpolate Oversampled Data.vi"("Bits of Precision Increase"=w479, "Waveform in"=w480) -> ("Waveform out"=w478:waveform(dbl))  [unwired: 9 in]
                n221 = call-poly <vilib>:"RMS.vi"("X"=w478) -> ("rms value"=w477:dbl)  [unwired: 1 out]
                n222 = Divide(x=w476, y=w477) -> (x/y=w475:dbl)
              }
            }
            n223 = Bundle By Name(cluster=w465, "Signal to noise ratio"=w462, "Signal to noise ratio (filtered)"=w463) -> (w464:T1)
          }
        }
      }
      frame Error {
        # "Error - Shutdown and display message"
        n224 = Generate User Event(user event=w486, event data cluster=User_Event_-_Enum."Shutdown" ("User Event - Enum")) -> ()  [unwired: 2 in, 2 out]
        n225 = call "DIHB DAQmx Task Name - Constant.vi"() -> ("DIHB DAQmx Task Name"=w482:string)  [unwired: 11 in]
        n226 = call <vilib>:"DAQmx Clear Task.vi"("task in"=w482) -> ()  [unwired: 14 in, 1 out]
      }
    }
  }
  n227 = while {
    shift-right: [w490] -> w15
    shift-left: w8 -> [w493]
    tunnel: w10 -> [w494]
    tunnel: w4 -> [w488]
    stop <- w491 stop-if-true
    # "This loop is the producer loop."
    n228 = event shown="[0] Panel Close;  Application Instance Close" {
      selector: w488 -> [_ _ _ _]
      dyn-events: _ -> [_ _ _ _]
      timeout: 50 -> [_ _ _ _]
      tunnel: w494 -> [w500 w507 _ w524]
      tunnel: w493 -> [w499 w508 w517 w526]
      tunnel: [w498 w506 w516 w525] -> w490
      tunnel: [FALSE ("stop") _ w515 _] -> w492
      event Panel Close; Application Instance Close {
        # "Front panel was closed, shutdown cleanly"
        n229 = event-data() -> ()  [unwired: 1 in, 2 out]
        n230 = Bundle By Name(cluster=T4 {"Program State"=enum."Calculate Velocity", "GUI Cluster"={"Sample Rate (Hz)"=2000000.0, "Number of Samples"=1000000, "Ready Button"=FALSE, "Filepath to Save Data"=path "", "Calibration File (TXT TSV)"=path "", "Interpolation (LP Filter)"=0.0}} ("element"), "Program State"=Program_State_-_Enum."Shutdown") -> (w495:T4)
        n231 = Enqueue Element(queue=w500, element=w495, error in (no error)=w499) -> (error out=w498:errorcluster)  [unwired: 1 in, 2 out]
      }
      event Timeout {
        n232 = event-data() -> ()  [unwired: 1 in, 2 out]
        n233 = Bundle By Name(cluster=T5 {"Sample Rate (Hz)"=2000000.0, "Number of Samples"=1000000, "Ready Button"=FALSE, "Filepath to Save Data"=path "", "Calibration File (TXT TSV)"=path "", "Interpolation (LP Filter)"=0.0} ("GUI State"), "Filepath to Save Data"="Filepath to Save Data (TSV)", "Calibration File (TXT TSV)"="Calibration File (TXT TSV)", "Sample Rate (Hz)"="Sample Rate (Hz)", "Number of Samples"="Number of Samples", "Interpolation (LP Filter)"="Interpolation (Low Pass Filter)") -> (w504:T5)
        n234 = Bundle By Name(cluster=T4 {"Program State"=enum."Calculate Velocity", "GUI Cluster"={"Sample Rate (Hz)"=2000000.0, "Number of Samples"=1000000, "Ready Button"=FALSE, "Filepath to Save Data"=path "", "Calibration File (TXT TSV)"=path "", "Interpolation (LP Filter)"=0.0}} ("input cluster"), "Program State"=Program_State_-_Enum."GUI Update", "GUI Cluster"=w504) -> (w503:T4)
        n235 = Enqueue Element(queue=w507, element=w503, error in (no error)=w508) -> (error out=w506:errorcluster)  [unwired: 1 in, 2 out]
      }
      event User Event {
        # "Consumer loop sent shutdown command"
        n236 = event-data() -> ("User Event - Enum"=w518:T2)  [unwired: 1 in]
        n237 = case shown="\"Shutdown\", Default" w518 {
          tunnel: w517 -> [w520]
          tunnel: [w520] -> w516
          tunnel: [TRUE ("stop")] -> w515
          frame "Shutdown", Default {
          }
        }
      }
      event "Ready Button": Value Change {
        n238 = event-data() -> ()  [unwired: 1 in, 2 out]
        n239 = Bundle By Name(cluster=T4 {"Program State"=enum."Calculate Velocity", "GUI Cluster"={"Sample Rate (Hz)"=2000000.0, "Number of Samples"=1000000, "Ready Button"=FALSE, "Filepath to Save Data"=path "", "Calibration File (TXT TSV)"=path "", "Interpolation (LP Filter)"=0.0}} ("input cluster"), "Program State"=Program_State_-_Enum."Make Ready") -> (w522:T4)
        n240 = Enqueue Element(queue=w524, element=w522, error in (no error)=w526) -> (error out=w525:errorcluster)  [unwired: 1 in, 2 out]
      }
    }
    n241 = Or(x=w490, y=w492) -> (x .or. y?=w491:bool)
  }
  n242 = Release Queue(queue=w10, error in (no error)=w15) -> (error out=w7:errorcluster)  [unwired: 1 in, 2 out]
  n243 = Merge Errors(w7, w6) -> (w5:errorcluster)
  n244 = call <vilib>:"Simple Error Handler.vi"("error in (no error)"=w5) -> ()  [unwired: 4 in, 5 out]
